vi "DAQMan TCP Control.vi"() -> ()   [LabVIEW 2012]
uses:
  <userlib>/STM/_SubVIs/stm_MetaDataElement.ctl
  <userlib>/STM/TCP/stm_TCP Read Options.ctl
  <userlib>/STM/TCP/STM Read Meta Data (TCP Ref).vi
  <userlib>/STM/TCP/STM Get Connection Reference (TCP).vi
  <userlib>/STM/TCP/STM Read Message (TCP).vi
  <userlib>/STM/TCP/STM Write Message (TCP).vi
panel:
  in  "Port":u16=5555
  out "Mode":string=" Run Mode 11:33 11/20/12"
  out "value":errorcluster
  out "Meta data":T1[](array[typedef])=["Mode", "AppError", "StartAcq", "StopAcq", "cDAQ1_Wfm", "cDAQ1_HSMetrics", "cDAQ1_Down", "cDAQ2_Wfm", "cDAQ2_HSMetrics", "cDAQ2_Down"]
  out "Updates":i32=44
  in  "client stop":bool
  in  "StartAcq":bool
  in  "StopAcq":bool
  in  "Target IP Address":string="localhost"
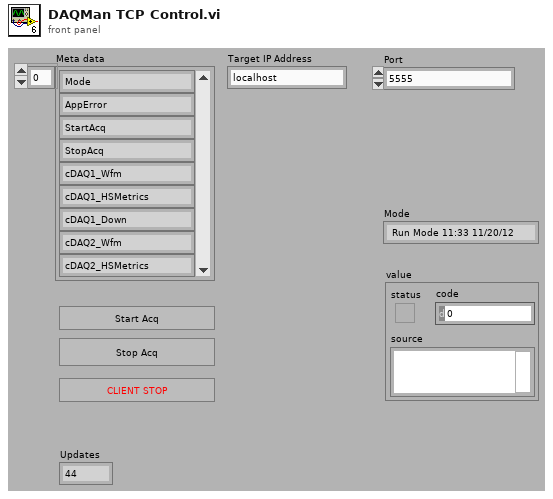
[diagram p1: front panel]
types:
  T1 = typedef "stm_MetaDataElement.ctl" = string
  T2 = typedef "stm_TCP Connection Info.ctl" = cluster{"connection ID":refnum<k5>, "Meta data":T1[]}
  T3 = typedef "stm_TCP Read Options.ctl" = cluster{"Ignore Timeout Error":bool, "timeout ms (1000)":i32}
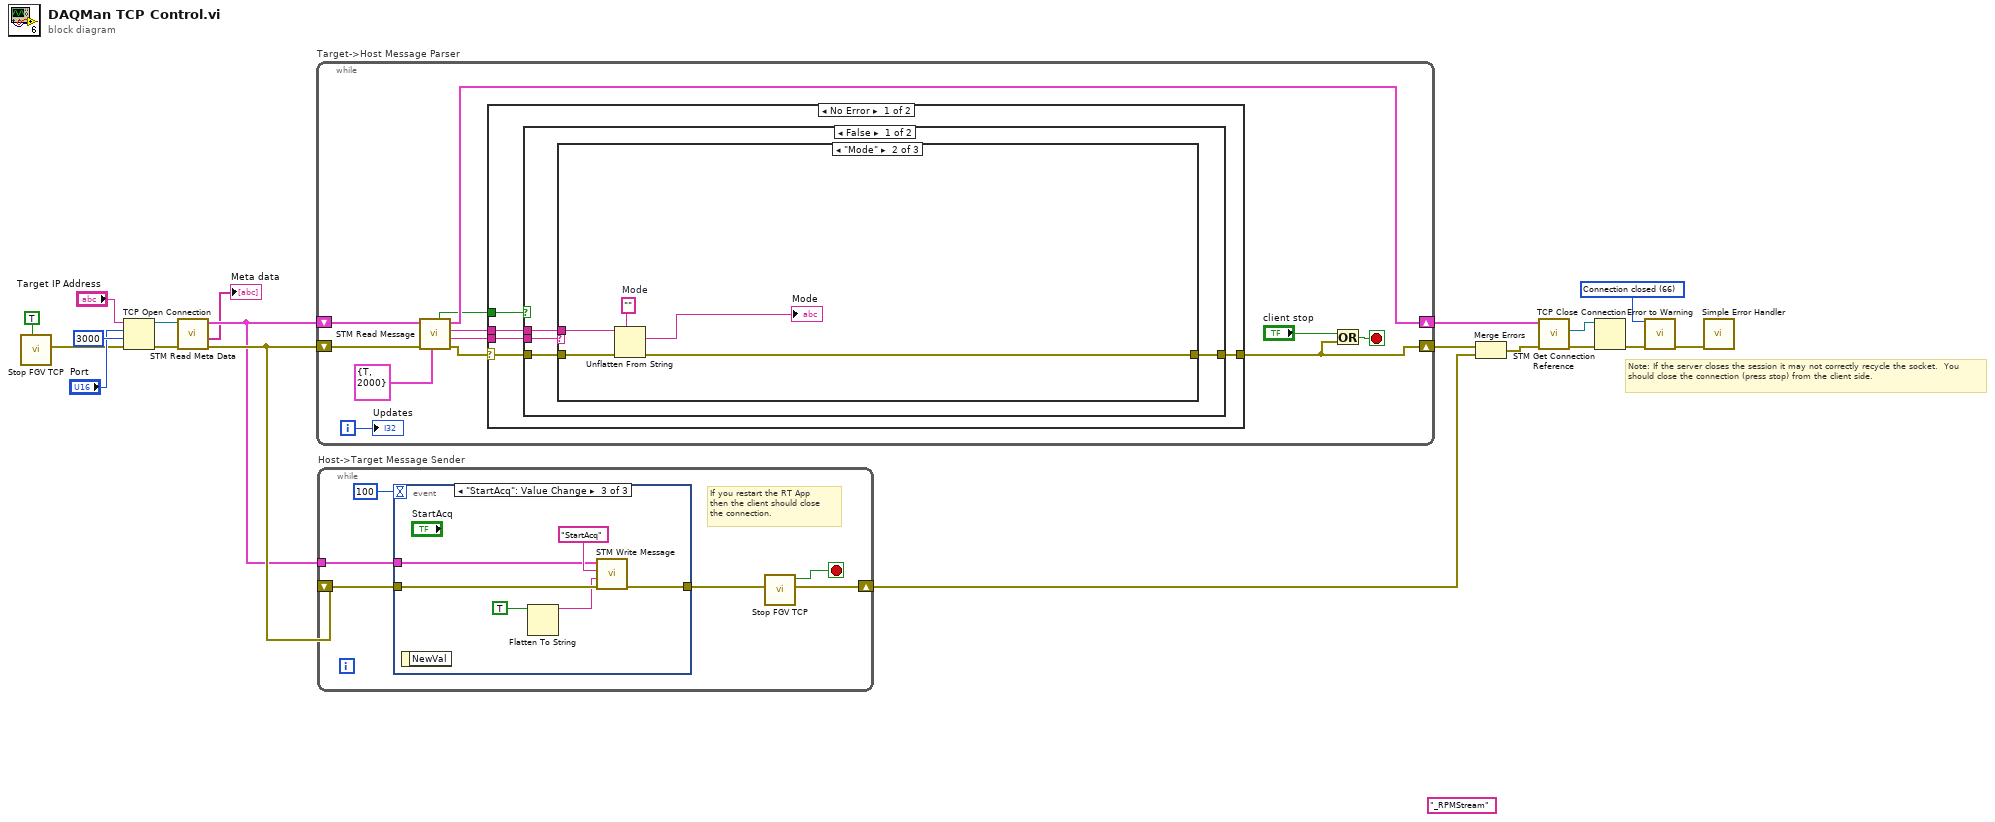
[diagram p0: block diagram]
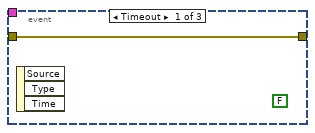
[diagram p2: hidden frame]
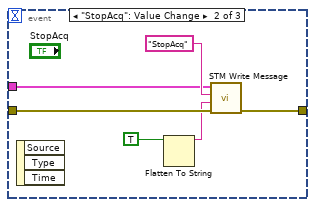
[diagram p3: hidden frame]
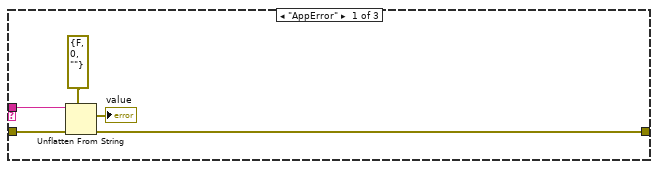
[diagram p4: hidden frame]
diagram:
  (unwired) "_RPMStream"
  w16 = 66 items=["No Error", "Argument Error", "Memory Full", "Out of Zone", "End of File", "File Already Open", "Generic File IO Error", "File Not Found", "File Permission Error", "Disk Full", "Duplicate Path", "Too Many Files Open", "Not Enabled", "Resource File Not Found", "Cannot Add Resource", "Resource Not Found", "Image Not Found", "Image Memory Error", "Pen Does Not Exist", "Config Bad Type", "Config Token Not Found", "Config Parse Error", "Config Memory Error", "Bad External Code Format", "Bad External Code Offset", "External Code Not Present", "Null Window", "Destroy Window Mixup", "Null Menu", "Print Aborted", "Bad Print Record", "Print Driver Error", "Windows Error During Print", "Memory Error During Print", "Print Dialog Error", "Generic Print Error", "Invalid Device Refnum", "Device Not Found", "Device Parameter Error", "Device Unit Error", "Can't Open Device", "Device Call Aborted", "Generic Error", "Cancelled By User", "Object ID Too Low", "Object ID Too High", "Object Not In Heap", "Unknown Heap", "Bad DefProc ID", "DefProc Not In Table", "Message Out Of Range", "Null Method", "Unknown Message", "Manager Call Not Supported", "Bad address", "Connection In progress", "Connection timed out", "Connection is already in progress", "Network attribute not supported", "Network error", "Address in use", "System out of memory", "Connection aborted", "Connection refused", "Connection is not connected", "Connection is already connected", "Connection closed", "Initialize error (interapplication manager)", "Bad occurrence", "Wait on unbound occurrence handler", "Occurrence queue overflow", "Bad path", "Semaphore not signaled", "Unrecognized type (interapplication manager)"] ("1st Error to Convert")
  # "Note: If the server closes the session it may not correctly recycle the socket.  You should close the connection (press stop) from the client side."
  n1 = call "Stop FGV TCP.vi"("Reset (F)"=TRUE) -> ("error out"=w2:errorcluster)  [unwired: 9 in, 1 out]
  n2 = TCP Open Connection(address="Target IP Address", remote port or service name="Port", timeout ms (60000)=3000, error in (no error)=w2) -> (connection ID=w19:refnum<k5>, error out=w18:errorcluster)  [unwired: 1 out]
  n3 = call-poly <userlib>:"STM Read Meta Data.vi"("error in"=w18, "connection ID"=w19) -> ("error out"=w8:errorcluster, "Meta data"=→"Meta data":T1[], "Connection Info Out"=w7:T2)  [unwired: 1 in, 6 out]
  n4 = while "Target->Host Message Parser" {
    shift-right: [w29] -> w15
    shift-left: w7 -> [w31]
    shift-right: [w20] -> w11
    shift-left: w8 -> [w30]
    i -> [w25]
    stop <- w22 stop-if-true
    n5 = call-poly <userlib>:"STM Read Message.vi"("Options"=T3 {"Ignore Timeout Error"=TRUE, "timeout ms (1000)"=2000}, "error in"=w30, "Connection Info"=w31) -> ("error out"=w26:errorcluster, "Name"=w24:T1, "data string"=w28:string, "Connection Info Out"=w29:T2, "Timed Out?"=w27:bool)  [unwired: 2 in, 2 out]
    n6 = case shown="No Error" w26 {
      selector: w26 -> [w34 w53]
      tunnel: w28 -> [w36 _]
      tunnel: w27 -> [w35 _]
      tunnel: [w33 w53] -> w20
      tunnel: w24 -> [w32 _]
      frame No Error {
        n7 = case shown="False" w35 {
          tunnel: w36 -> [w40 _]
          tunnel: w34 -> [w39 w52]
          tunnel: [w38 w52] -> w33
          tunnel: w32 -> [w37 _]
          frame False {
            n8 = case shown="\"Mode\"" w37 {
              tunnel: w40 -> [w43 w49 _]
              tunnel: w39 -> [w45 w50 w51]
              tunnel: [w42 w48 w51] -> w38
              frame "AppError" {
                n9 = Unflatten From String(type=errorcluster {"status"=FALSE, "code"=0, "source"=""} ("error in (no error)"), binary string=w43, error in (no error)=w45) -> (value=→"value":errorcluster, error out=w42:errorcluster)  [unwired: 3 out]
              }
              frame "Mode" {
                w47 = ""  # Mode
                n10 = Unflatten From String(type=w47, binary string=w49, error in (no error)=w50) -> (value=→"Mode":string, error out=w48:errorcluster)  [unwired: 3 out]
              }
              frame Default {
              }
            }
          }
          frame True {
          }
        }
      }
      frame Error {
      }
    }
    n11 = Or(x="client stop", y=w20) -> (x .or. y?=w22:bool)
    "Updates" <- w25
  }
  n12 = while "Host->Target Message Sender" {
    tunnel: w7 -> [w59]
    shift-right: [w55] -> w12
    shift-left: w8 -> [w58]
    stop <- w54 stop-if-true
    # "If you restart the RT App\nthen the client should close\nthe connection."
    n13 = event shown="[2] \"StartAcq\": Value Change" {
      selector: _ -> [_ _ _]
      dyn-events: _ -> [_ _ _]
      timeout: 100 -> [_ _ _]
      tunnel: w59 -> [_ w65 w70]
      tunnel: w58 -> [w60 w64 w71]
      tunnel: [w60 w61 w69] -> w56
      event Timeout {
        (unwired) FALSE ("stop")
        n14 = event-data() -> ()  [unwired: 4 out]
      }
      event "StopAcq": Value Change {
        n15 = event-data() -> ()  [unwired: 4 out]
        n16 = Flatten To String(anything=TRUE ("stop")) -> (data string=w63:string)  [unwired: 2 in, 3 out]
        n17 = call-poly <userlib>:"STM Write Message.vi"("error in (no error)"=w64, "Data"=w63, "Name"="StopAcq", "Connection Info"=w65) -> ("error out"=w61:errorcluster)  [unwired: 1 in, 6 out]
      }
      event "StartAcq": Value Change {
        n18 = event-data() -> ()  [unwired: 2 out]
        n19 = Flatten To String(anything=TRUE ("Force Trig")) -> (data string=w68:string)  [unwired: 2 in, 3 out]
        n20 = call-poly <userlib>:"STM Write Message.vi"("error in (no error)"=w71, "Data"=w68, "Name"="StartAcq", "Connection Info"=w70) -> ("error out"=w69:errorcluster)  [unwired: 1 in, 6 out]
      }
    }
    n21 = call "Stop FGV TCP.vi"("error in"=w56) -> ("error out"=w55:errorcluster, "Stop?"=w54:bool)  [unwired: 9 in]
  }
  n22 = Merge Errors(w11, w12) -> (w10:errorcluster)
  n23 = call-poly <userlib>:"STM Get Connection Reference.vi"("error in"=w10, "Connection Info"=w15) -> ("error out"=w13:errorcluster, "connection ID out"=w14:refnum<k5>)  [unwired: 8 out]
  n24 = TCP Close Connection(connection ID=w14, error in (no error)=w13) -> (error out=w9:errorcluster)  [unwired: 2 out]
  n25 = call <vilib>:"Error to Warning.vi"("1st Error to Convert"=w16, "error in"=w9) -> ("warning out"=w6:errorcluster)  [unwired: 3 in, 10 out]
  n26 = call <vilib>:"Simple Error Handler.vi"("error in (no error)"=w6) -> ()  [unwired: 4 in, 5 out]
